vi "WriteCSV.vi"(2 "session in":refnum<k35>, 3 "Signal":dbl[](array[numeric]) format="%#_13g", 4 "NumericData":dbl[](array[numeric]) format="%#_13g", 5 "StringData":string[](array[string])) -> (0 "session out":refnum<k35>, 1 "Error Message":string)   [LabVIEW 2018]
panel:
  in  "Script Path":path=path "C:/Users/Ptgroup/Documents/UVA-Lab-Software/LANL-System/rssmt/Python_Files/db.py"
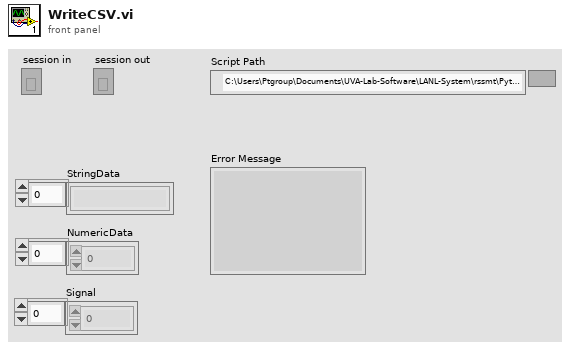
[diagram p1: front panel]
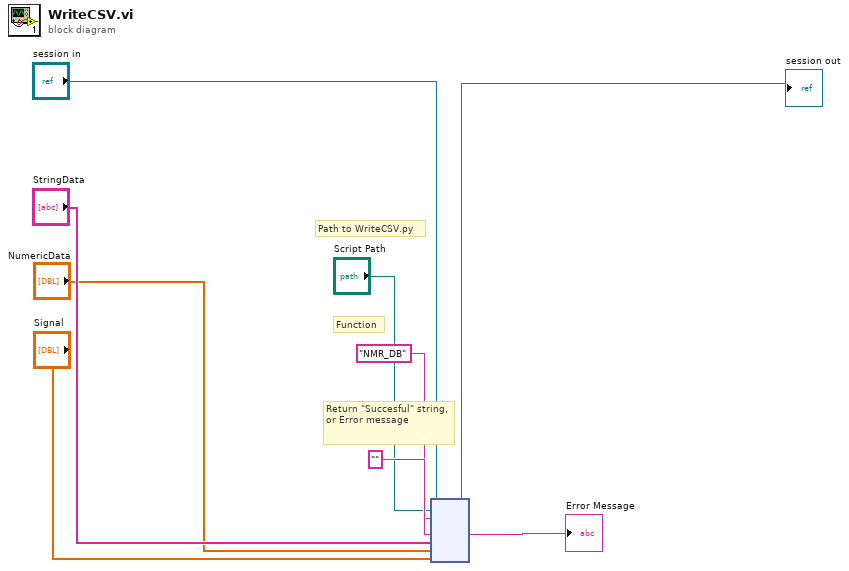
[diagram p0: block diagram]
diagram:
  # "Path to WriteCSV.py"
  # "Function"
  # "Return \"Succesful\" string, or Error message"
  n1 = node("session in", "Script Path", "NMR_DB" ("function name"), "", "StringData", "NumericData", "Signal") -> (→"session out":refnum<k35>, →"Error Message":string)  [unwired: 4 in, 3 out]
